vi "File Path to String.vi"(8 "error in":errorcluster, 11 "MPLab in":refnum<class "MPLab.lvclass">) -> (0 "error out":errorcluster, 3 "MPLab out":refnum<class "MPLab.lvclass">)   [LabVIEW 2018, in "MPLab.lvlib" / "MPLab.lvclass"]
uses:
  MPLab.lvclass
  MPLab.lvclass/MPLab.ctl
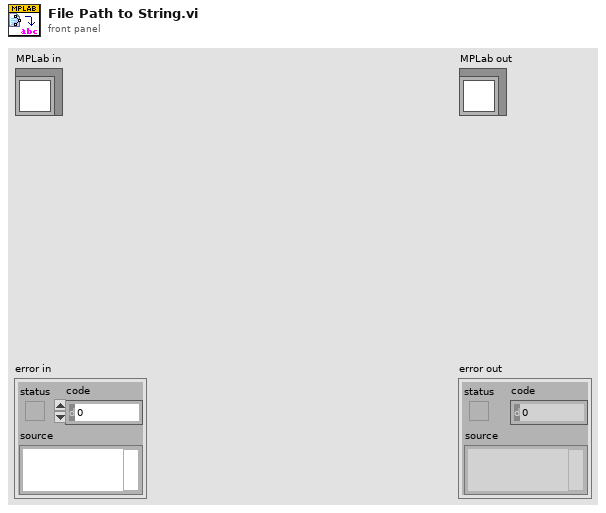
[diagram p1: front panel]
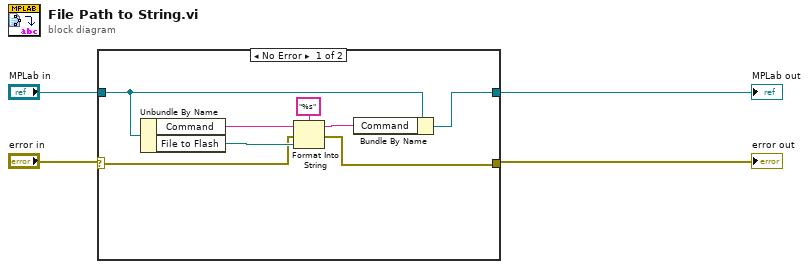
[diagram p0: block diagram]
diagram:
  n1 = case shown="No Error" "error in" {
    selector: "error in" -> [w5 w14]
    tunnel: [w10 w14] -> w4
    tunnel: "MPLab in" -> [w9 w13]
    tunnel: [w8 w13] -> w2
    frame No Error {
      n2 = Unbundle By Name(w9) -> ("Command"=w11:string, "File to Flash"=w12:path)
      n3 = Format Into String(format string="%s" ("string"), initial string=w11, error in=w5, w12) -> (resulting string=w7:string, error out=w10:errorcluster)
      n4 = Bundle By Name(cluster=w9, "Command"=w7) -> (w8:refnum<class "MPLab.lvclass">)
    }
    frame Error {
    }
  }
  "error out" <- w4
  "MPLab out" <- w2
